vi "format into Sonde Data Array.vi"(11 "data":string[][](array[string])) -> (3 "Array":string[][](array[string]))   [LabVIEW 2016]
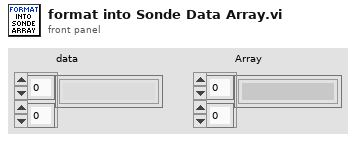
[diagram p1: front panel]
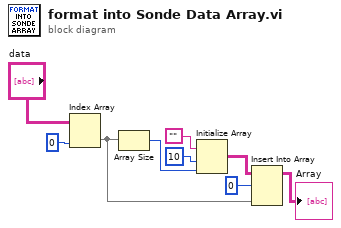
[diagram p0: block diagram]
diagram:
  n1 = Index Array(array="data", index (col)=0 ("disabled index (col)")) -> (element=w8:string[])  [unwired: 1 in]
  n2 = Array Size(array=w8) -> (size(s)=w1:i32)
  n3 = Initialize Array("", 10 ("dimension size"), w1) -> (w3:string[][])
  n4 = Insert Into Array(array=w3, index (row)=0, new element=w8) -> (→"Array":string[][])  [unwired: 1 in]
